vi "Get Right Pot Value.vi"(11 "drive.lvclass":refnum<class "drive.lvclass">) -> (2 "Value":dbl, 3 "drive.lvclass":refnum<class "drive.lvclass">)   [LabVIEW 2015, in "drive.lvclass"]
uses:
  drive.lvclass
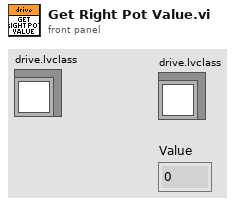
[diagram p1: front panel]
types:
  T1 = typedef "WPI_PotentiometerDevRef.ctl" = cluster{"DevStatus":errorcluster, "Analog Channel":T2, "Invert Output":bool}
  T2 = typedef "FPGA_AIChannel.ctl" = enum8{"AI 0", "AI 1", "AI 2", "AI 3", "AI MXP 0", "AI MXP 1", "AI MXP 2", "AI MXP 3", "Invalid"}
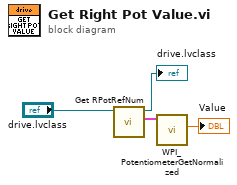
[diagram p0: block diagram]
diagram:
  n1 = call-dynamic "Get RPotRefNum.vi"("drive in"="drive.lvclass") -> ("PotDevRef"=w2:T1, "drive out"=→"drive.lvclass":refnum<class "drive.lvclass">)  [unwired: 8 in, 1 out]
  n2 = call <vilib>:"WPI_PotentiometerGetNormalized.vi"("PotDevRef"=w2) -> ("Normalized Value"=→"Value":dbl)  [unwired: 8 in, 2 out]
